vi "Interpolate_Curve.vi"(4 "Cursor List":T3, 6 "uTTA_MetaData_in":T1 {"No Suspect Lines" format="%.3pV"; "Interpolation Factor m" format="%.2g"; "Interpolation Offset" format="%.2g"; "Chip Size" format="%.2gmm²"; "Heating Power" format="%.3pW"; "Cool Volt Deviation" format="%.3pV"; "Cool Voltage" format="%.3pV"; "Tsamp,fast" format="%#_3gus"; "Tsamp,slow" format="%#_3gus"; "T_Preheat" format="%#_3gs"; "T_Heat" format="%#_3gs"; "T_Cool" format="%#_3gs"}, 7 "uTTA_MeasData_in":T2, 8 "First Samples":i32, 9 "PlotScale [SQRT-Sclale]":bool) -> (0 "uTTA_MetaData_out":T1 {"No Suspect Lines" format="%.3pV"; "Interpolation Factor m" format="%.2g"; "Interpolation Offset" format="%.2g"; "Chip Size" format="%.2gmm²"; "Heating Power" format="%.3pW"; "Cool Volt Deviation" format="%.3pV"; "Cool Voltage" format="%.3pV"; "Tsamp,fast" format="%#_3gus"; "Tsamp,slow" format="%#_3gus"; "T_Preheat" format="%#_3gs"; "T_Heat" format="%#_3gs"; "T_Cool" format="%#_3gs"}, 1 "uTTA_MeasData_out":T2, 3 "Plot":cluster{dbl[], dbl[]}[](array[cluster]))   [LabVIEW 2021]
uses:
  <vilib>/Utility/miscctls.llb/LVCursorListTypeDef.ctl
  uTTA_MetaData.ctl
  CTL_uTTA_MeasurementData.ctl
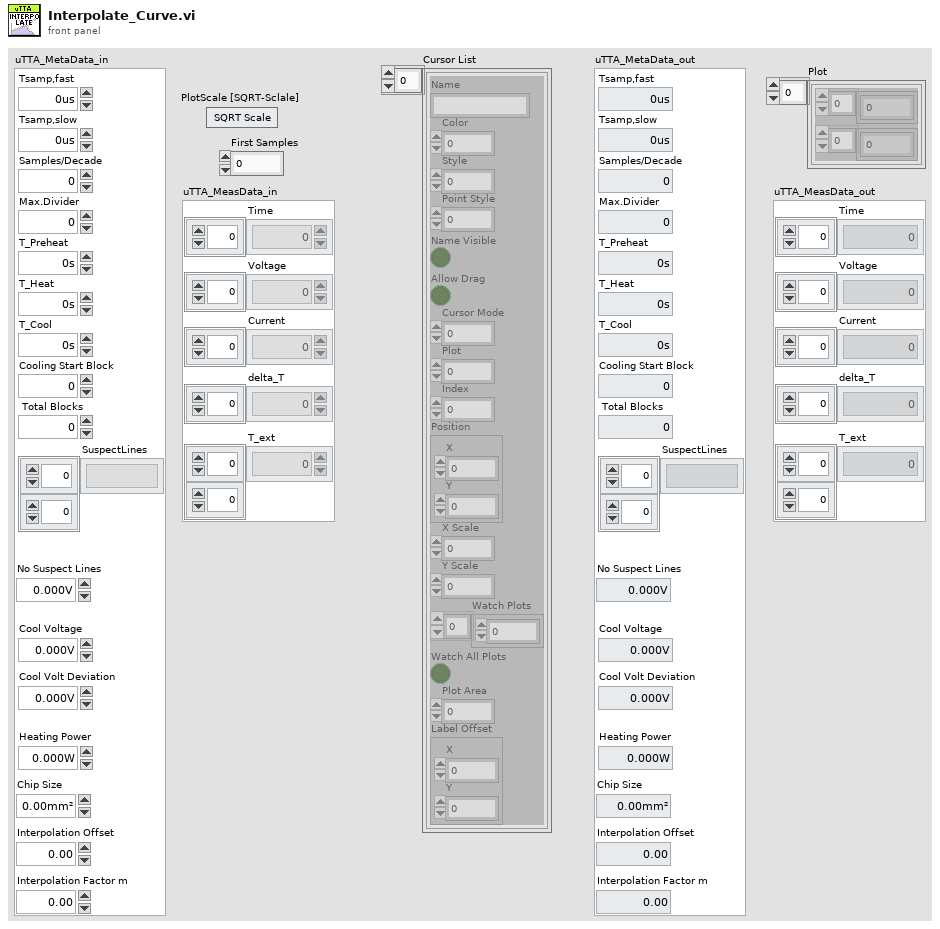
[diagram p1: front panel]
types:
  T1 = typedef "uTTA_MetaData.ctl" = cluster{"Tsamp,fast":dbl, "Tsamp,slow":dbl, "Samples/Decade":u32, "Max.Divider":u32, "T_Preheat":dbl, "T_Heat":dbl, "T_Cool":dbl, "Cooling Start Block":u32, " Total Blocks":u32, "SuspectLines":string[][], "Cool Voltage":dbl, "Cool Volt Deviation":dbl, "Heating Power":dbl, "Chip Size":dbl, "Interpolation Offset":dbl, "Interpolation Factor m":dbl, "No Suspect Lines":u32}
  T2 = typedef "CTL_uTTA_MeasurementData.ctl" = cluster{"Time":dbl[], "Voltage":dbl[], "Current":dbl[], "delta_T":dbl[], "T_ext":dbl[][]}
  T3 = typedef "LVCursorListTypeDef.ctl" = cluster{"Name":string, "Color":u32, "Style":u8, "Point Style":u8, "Name Visible":bool, "Allow Drag":bool, "Cursor Mode":u32, "Plot":i32, "Index":i32, "Position":cluster{"X":dbl, "Y":dbl}, "X Scale":u32, "Y Scale":u32, "Watch Plots":i32[], "Watch All Plots":bool, "Plot Area":i32, "Label Offset":cluster{"X":dbl, "Y":dbl}}[]
  T4 = cluster{"Name":string, "Color":u32, "Style":u8, "Point Style":u8, "Name Visible":bool, "Allow Drag":bool, "Cursor Mode":u32, "Plot":i32, "Index":i32, "Position":cluster{"X":dbl, "Y":dbl}, "X Scale":u32, "Y Scale":u32, "Watch Plots":i32[], "Watch All Plots":bool, "Plot Area":i32, "Label Offset":cluster{"X":dbl, "Y":dbl}}
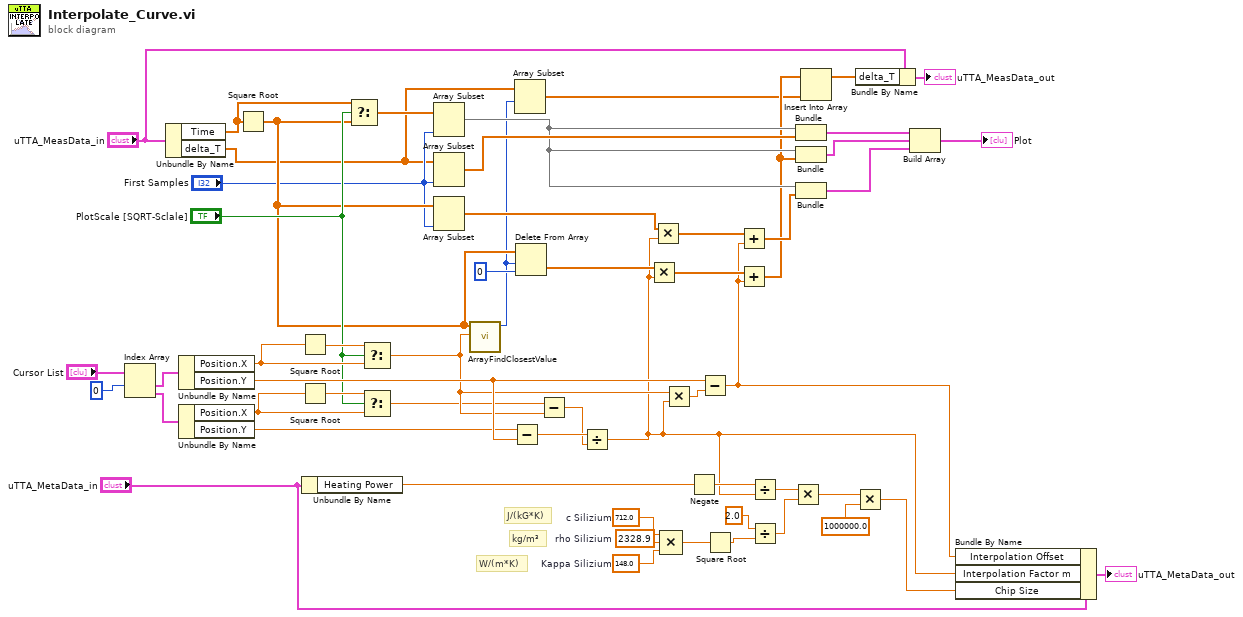
[diagram p0: block diagram]
diagram:
  w40 = 148.0  # Kappa Silizium
  w39 = 2328.9  # rho Silizium
  w38 = 712.0  # c Silizium
  # "W/(m*K)"
  # "kg/m³"
  # "J/(kG*K)"
  n1 = Index Array(array="Cursor List", index #1=0 ("index")) -> (element #1=w28:T4, element #2=w27:T4)  [unwired: 1 in]
  n2 = Unbundle By Name("uTTA_MeasData_in") -> ("Time"=w11:dbl[], "delta_T"=w10:dbl[])
  n3 = Unbundle By Name(w28) -> ("Position.X"=w24:dbl, "Position.Y"=w50:dbl)
  n4 = Unbundle By Name(w27) -> ("Position.X"=w20:dbl, "Position.Y"=w37:dbl)
  n5 = Square Root(x=w11) -> (sqrt(x)=w17:dbl[])
  n6 = Square Root(x=w24) -> (sqrt(x)=w25:dbl)
  n7 = Square Root(x=w20) -> (sqrt(x)=w21:dbl)
  n8 = Unbundle By Name("uTTA_MetaData_in") -> ("Heating Power"=w6:dbl)
  n9 = Select(t=w11, s="PlotScale [SQRT-Sclale]", f=w17) -> (s? t:f=w26:dbl[])
  n10 = Select(t=w25, s="PlotScale [SQRT-Sclale]", f=w24) -> (s? t:f=w23:dbl)
  n11 = Select(t=w21, s="PlotScale [SQRT-Sclale]", f=w20) -> (s? t:f=w22:dbl)
  n12 = Array Subset(array=w26, length="First Samples") -> (w18:dbl[])  [unwired: 1 in]
  n13 = Array Subset(array=w10, length="First Samples") -> (w33:dbl[])  [unwired: 1 in]
  n14 = Array Subset(array=w17, length="First Samples") -> (w15:dbl[])  [unwired: 1 in]
  n15 = call "ArrayFindClosestValue.vi"("Search Item"=w23, "Array"=w17) -> ("Index"=w14:i32)  [unwired: 9 in]
  n16 = Subtract(x=w37, y=w50) -> (x-y=w48:dbl)
  n17 = Array Subset(array=w10, index=w14) -> (w12:dbl[])  [unwired: 1 in]
  n18 = Delete From Array(array=w17, length=w14, index=0) -> (deleted portion=w31:dbl[])  [unwired: 1 out]
  n19 = Subtract(x=w22, y=w23) -> (x-y=w32:dbl)
  n20 = Divide(x=w48, y=w32) -> (x/y=w3:dbl)
  n21 = Multiply(x=w31, y=w3) -> (x*y=w53:dbl[])
  n22 = Multiply(x=w15, y=w3) -> (x*y=w54:dbl[])
  n23 = Compound Arithmetic op=MULTIPLY(w38, w39, w40) -> (w44:dbl)
  n24 = Multiply(x=w23, y=w3) -> (x*y=w49:dbl)
  n25 = Negate(x=w6) -> (-x=w51:dbl)
  n26 = Subtract(x=w50, y=w49) -> (x-y=w2:dbl)
  n27 = Square Root(x=w44) -> (sqrt(x)=w43:dbl)
  n28 = Add(x=w54, y=w2) -> (x+y=w55:dbl[])
  n29 = Add(x=w53, y=w2) -> (x+y=w13:dbl[])
  n30 = Divide(x=w51, y=w3) -> (x/y=w41:dbl)
  n31 = Divide(x=2.0, y=w43) -> (x/y=w45:dbl)
  n32 = Multiply(x=w41, y=w45) -> (x*y=w47:dbl)
  n33 = Bundle(w18, w33) -> (w35:cluster{dbl[], dbl[]})  [unwired: 1 in]
  n34 = Bundle(w18, w13) -> (w36:cluster{dbl[], dbl[]})  [unwired: 1 in]
  n35 = Bundle(w18, w55) -> (w56:cluster{dbl[], dbl[]})  [unwired: 1 in]
  n36 = Insert Into Array(array=w13, new element=w12) -> (w8:dbl[])  [unwired: 1 in]
  n37 = Multiply(x=w47, y=1000000.0) -> (x*y=w4:dbl)
  n38 = Bundle By Name(cluster="uTTA_MeasData_in", "delta_T"=w8) -> (→"uTTA_MeasData_out":T2)
  n39 = Build Array(w35, w36, w56) -> (→"Plot":cluster{dbl[], dbl[]}[])
  n40 = Bundle By Name(cluster="uTTA_MetaData_in", "Interpolation Offset"=w2, "Interpolation Factor m"=w3, "Chip Size"=w4) -> (→"uTTA_MetaData_out":T1)
